vi "Channel_Rename_Array.vi"(1 "通道数量":u8) -> (0 "通道名称":string[](array[string]))   [LabVIEW 2018]
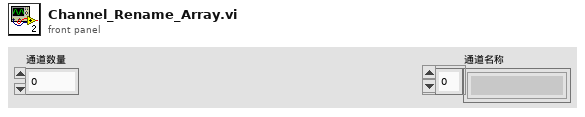
[diagram p1: front panel]
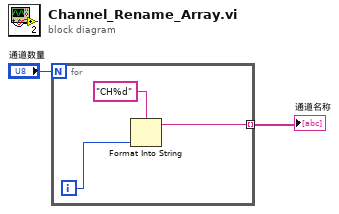
[diagram p0: block diagram]
diagram:
  n1 = for {
    N: "通道数量" -> [_]
    tunnel: [w4] -> w2 mode=indexing
    i -> [w3]
    n2 = Format Into String(format string="CH%d" ("格式字符串"), w3) -> (resulting string=w4:string)  [unwired: 2 in, 1 out]
  }
  "通道名称" <- w2
